vi "interp1.vi"(0 "X":dbl[](array[numeric]), 2 "Y":dbl[](array[numeric]), 3 "U":dbl, 4 "extrapolate":bool) -> (5 "V":dbl)   [LabVIEW 2020]
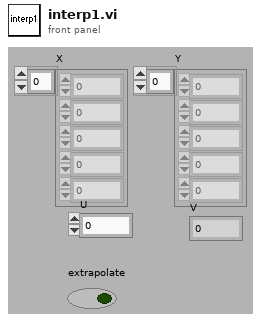
[diagram p1: front panel]
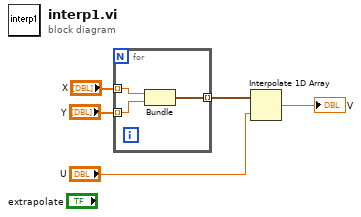
[diagram p0: block diagram]
diagram:
  n1 = for {
    tunnel: "X" -> [w8] mode=indexing
    tunnel: "Y" -> [w7] mode=indexing
    tunnel: [w6] -> w3 mode=indexing
    n2 = Bundle("Numeric"=w8, "Numeric"=w7) -> (w6:cluster{"Numeric":dbl, "Numeric":dbl})  [unwired: 1 in]
  }
  n3 = Interpolate 1D Array(1:"U", 2:w3) -> (0:→"V":dbl)
